vi "Check1DStringArrayForDuplicates.vi"(11 "String Array":string[](array[string])) -> (3 "duplicate string found?":bool)   [LabVIEW 2012]
doc: "Sort the input string array, make a copy, and delete the first element.\nThe array with the element deleted is compared against the complete array (note that both arrays are sorted)\nIf there are no duplicates, a match between the 2 arrays should NOT occur"
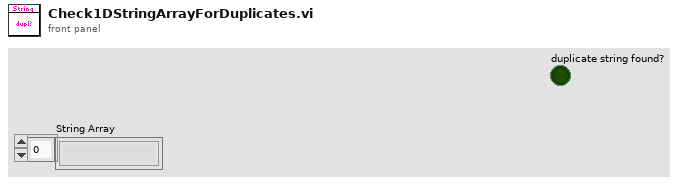
[diagram p1: front panel]
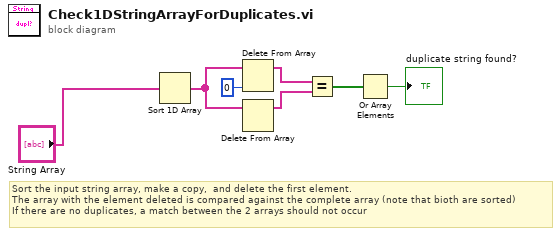
[diagram p0: block diagram]
diagram:
  # "Sort the input string array, make a copy,  and delete the first element.\nThe array with the element deleted is compared against the complete array (note that bioth are sorted)\nIf there are no duplicates, a match between the 2 arrays should not occur"
  n1 = Sort 1D Array(array="String Array") -> (sorted array=w7:string[])
  n2 = Delete From Array(array=w7, index=0) -> (array with subset deleted=w5:string[])  [unwired: 1 in, 1 out]
  n3 = Delete From Array(array=w7) -> (array with subset deleted=w4:string[])  [unwired: 2 in, 1 out]
  n4 = Equal?(x=w5, y=w4) -> (x = y?=w3:bool[])
  n5 = Or Array Elements(Boolean array=w3) -> (logical OR=→"duplicate string found?":bool)
